vi "Handle Windows Errors.vi"(8 "error in (no error)":errorcluster, 11 "Handle":i64) -> (0 "error out":errorcluster)   [LabVIEW 2015, in "Simple Progress Bar.lvlib"]
uses:
  Simple Progress Bar.lvlib
  <vilib>/Utility/error.llb/Error Cluster From Error Code.vi
  <vilib>/ErrorRing/Error Ring.xnode
  kernel32.dll
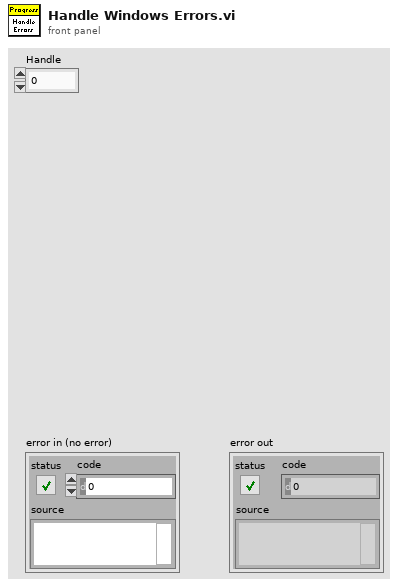
[diagram p1: front panel]
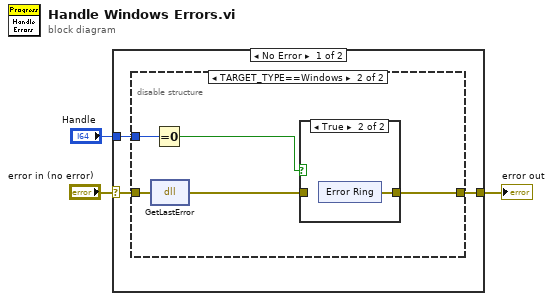
[diagram p0: block diagram]
diagram:
  n1 = case shown="No Error" "error in (no error)" {
    selector: "error in (no error)" -> [w6 w20]
    tunnel: [w5 w20] -> w2
    tunnel: "Handle" -> [w4 _]
    frame No Error {
      n2 = disable-structure shown="TARGET_TYPE==Windows" {
        disable-tunnel: w6 -> [w7 w11]
        disable-tunnel: [w7 w8] -> w5
        disable-tunnel: w4 -> [_ w12]
        frame condition #0 {
          # "#ToError"
        }
        frame condition #1 (active) {
          n3 = dll-call lib="kernel32.dll" fn="GetLastError"(error in=w11) -> (error out=w9:errorcluster)  [unwired: 3 in, 1 out]
          n4 = Equal To 0?(x=w12) -> (x = 0?=w10:bool)
          n5 = case shown="True" w10 {
            tunnel: [w13 w14] -> w8
            tunnel: w9 -> [w13 _]
            frame False {
            }
            frame True {
              n6 = xnode "Error Ring"() -> ("error out"=w14:errorcluster)
            }
          }
        }
      }
    }
    frame Error {
    }
  }
  "error out" <- w2
